vi "Global_MicroscopeView.vi"(2 "Image Type":T1 items=["Grayscale (U8)", "Grayscale (I16)", "Grayscale (SGL)", "Complex (CSG)", "RGB (U32)", "HSL (U32)", "RGB (U64)", "Grayscale (U16)"], 3 "Initialise":bool, 4 "New Image":T2, 5 "Update Image":bool) -> (0 "error out":errorcluster, 1 "MicroscopeView":T2)   [LabVIEW 2015]
uses:
  <vilib>/vision/Image Controls.llb/IMAQ Image.ctl
panel:
  in  "Times executed":dbl
  in  "last saved time":u32
  # "Internal counter"
  # "INPUTS"
  # "OUTPUTS"
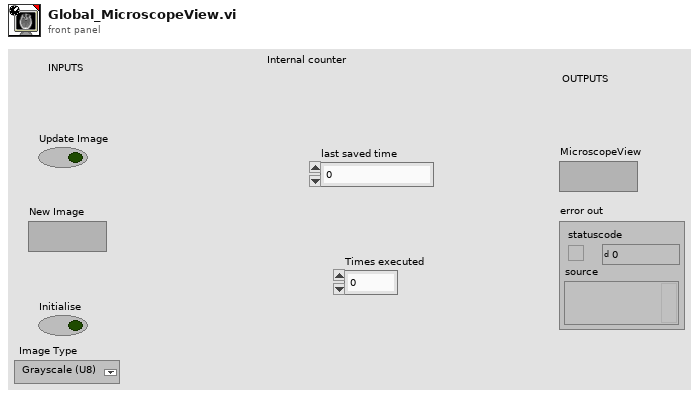
[diagram p1: front panel]
types:
  T1 = typedef "Image Type" = u32
  T2 = typedef "IMAQ Image.ctl" = refnum<image>
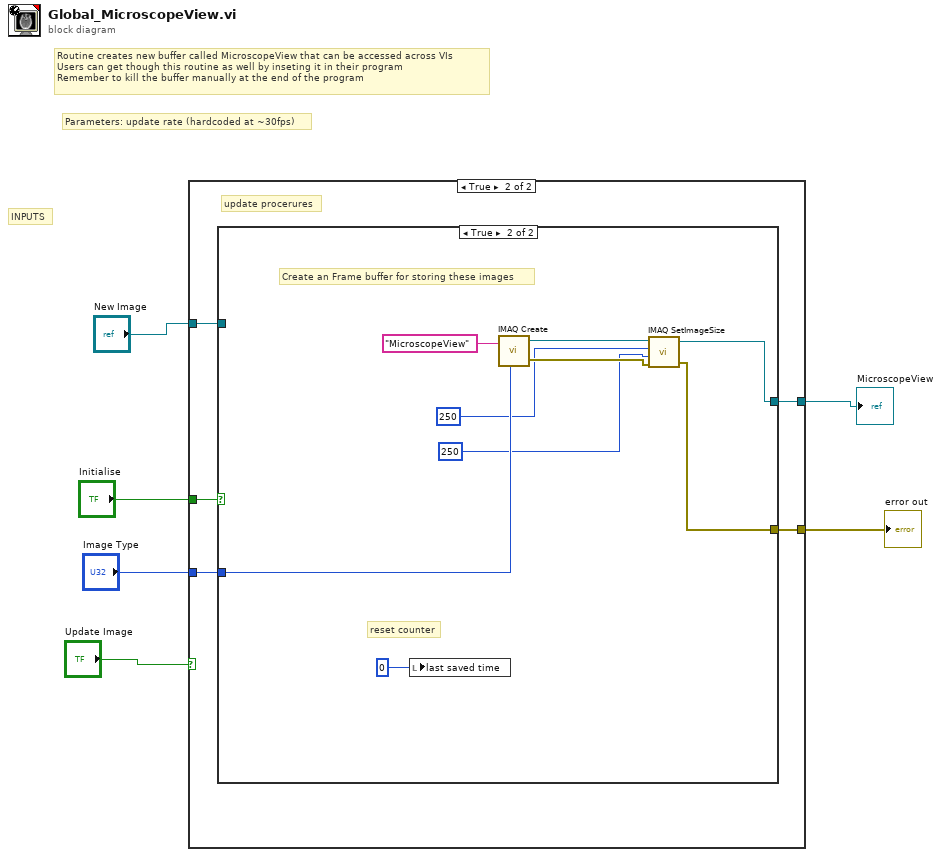
[diagram p0: block diagram]
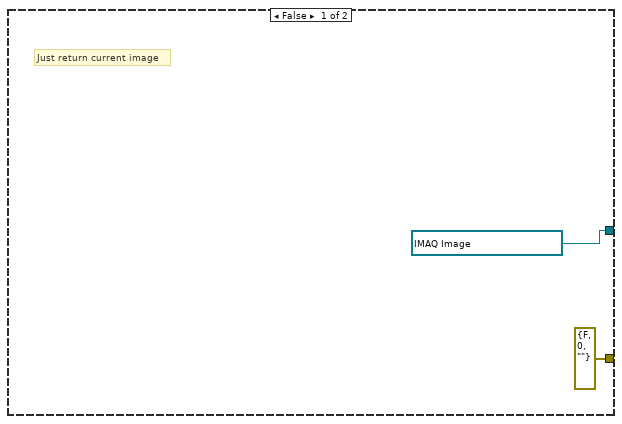
[diagram p2: hidden frame]
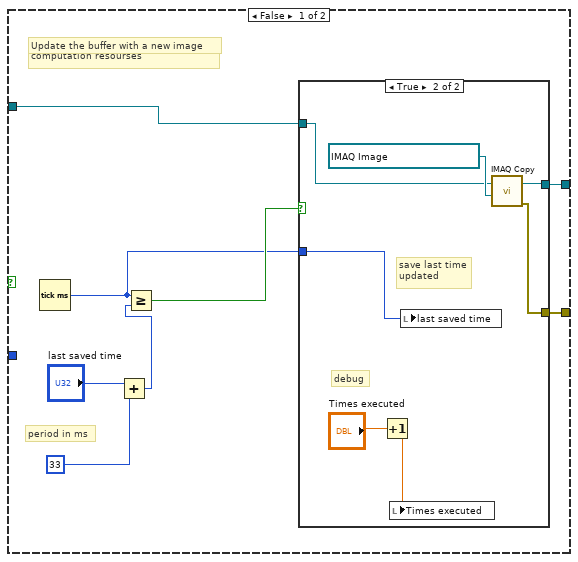
[diagram p3: hidden frame]
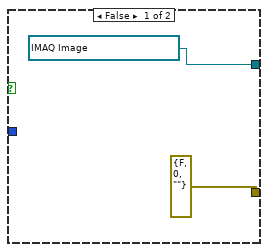
[diagram p4: hidden frame]
diagram:
  # "Parameters: update rate (hardcoded at ~30fps)"
  # "Routine creates new buffer called MicroscopeView that can be accessed across VIs\nUsers can get though this routine as well by inseting it in their program\nRemember to kill the buffer manually at the end of the program"
  # "INPUTS"
  n1 = case shown="True" "Update Image" {
    tunnel: [T2 refnum ("Image") w13] -> w6
    tunnel: "New Image" -> [_ w12]
    tunnel: [errorcluster {"status"=FALSE, "code"=0, "source"=""} ("error out") w11] -> w4
    tunnel: "Image Type" -> [_ w10]
    tunnel: "Initialise" -> [_ w9]
    frame False {
      # "Just return current image"
    }
    frame True {
      # "update procerures"
      n2 = case shown="True" w9 {
        tunnel: [w21 w35] -> w13
        tunnel: w12 -> [w20 _]
        tunnel: [w19 w36] -> w11
        tunnel: w10 -> [_ w38]
        frame False {
          # "period in ms"
          # "update at limited frame rate to save\ncomputation resourses"
          # "Update the buffer with a new image"
          n3 = Tick Count (ms)() -> (millisecond timer value=w14:u32)
          n4 = Add(x="last saved time", y=u32 33) -> (x+y=w16:u32)
          n5 = Greater Or Equal?(x=w14, y=w16) -> (x >= y?=w15:bool)
          n6 = case shown="True" w15 {
            tunnel: [T2 refnum ("Image") w30] -> w21
            tunnel: w20 -> [_ w24]
            tunnel: [errorcluster {"status"=FALSE, "code"=0, "source"=""} ("error out") w29] -> w19
            tunnel: w14 -> [_ w28]
            frame False {
            }
            frame True {
              # "debug"
              # "save last time\nupdated"
              n7 = Increment(x="Times executed") -> (x+1=w26:dbl)
              n8 = local write "Times executed"(w26) -> ()
              n9 = local write "last saved time"(w28) -> ()
              n10 = call "IMAQ Copy"("Image Dst"=T2 refnum ("Image"), "Image Src"=w24) -> ("error out"=w29:errorcluster, "Image Dst Out"=w30:T2)  [unwired: 4 in]
            }
          }
        }
        frame True {
          # "reset counter"
          # "Create an Frame buffer for storing these images"
          n11 = local write "last saved time"(u32 0 ("last saved time")) -> ()
          n12 = call "IMAQ Create"("Image Name"="MicroscopeView", "Image Type"=w38) -> ("New Image"=w34:T2, "error out"=w33:errorcluster)  [unwired: 3 in]
          n13 = call "IMAQ SetImageSize"("error in (no error)"=w33, "Y Resolution"=250 ("X Resolution"), "X Resolution"=250, "Image"=w34) -> ("error out"=w36:errorcluster, "Image Out"=w35:T2)  [unwired: 1 in]
        }
      }
    }
  }
  "MicroscopeView" <- w6
  "error out" <- w4
